vi "SISO-State-Space-Model-01.vi"() -> ()   [LabVIEW 2022 SP3]
uses:
  <vilib>/addons/System Identification/Model Typedefs.llb/si_Bode Magnitude Plot.ctl
  <vilib>/addons/System Identification/Model Typedefs.llb/si_Bode Phase Plot.ctl
  <vilib>/Utility/file.llb/Read Delimited Spreadsheet (DBL).vi
  <vilib>/addons/System Identification/Frequency Domain Estimation.llb/SI Estimate Discrete Transfer Function Model from FRF (SISO Arbitrary).vi
  <vilib>/addons/System Identification/NI_SysID.lvlib
  <vilib>/addons/System Identification/Frequency Domain Estimation.llb/SI Estimate Discrete State-Space Model from FRF (SISO Arbitrary).vi
  <vilib>/Analysis/NI_AALPro.lvlib
  <vilib>/Analysis/6fits.llb/Confidence Interval (Gauss).vi
  <vilib>/Analysis/6fits.llb/Confidence Interval (Power).vi
  <vilib>/Analysis/6fits.llb/Confidence Interval (Log).vi
  <vilib>/Analysis/6fits.llb/Confidence Interval (Exp).vi
  <vilib>/Analysis/6fits.llb/Confidence Interval (Linear).vi
panel:
  out "Bode phase plot":T1
  out "Bode magnitude plot":T2
  in  "freq info":T3={"start frequency"=-1.0, "end frequency"=-1.0, "num of freq bins"=1000, "interval type"=0} {"interval type" items=["logarithmic", "linear"]; "end frequency" format="%.2f"; "start frequency" format="%.2f"}
  in  "orders of transfer function model":cluster{" num order":i32, "den order":i32}={" num order"=1, "den order"=2}
  out "Observed Data and Fitted Curve":cluster{cluster{dbl, "Numeric":dbl}[]}[](graph)
  in  "Data Set":T4(ring)
  in  "Tolerance":dbl=0.0001
  in  "Fitting Method":u16(ring) items=["Least Square", "Least Absolute Residual", "Bisquare"]
  out "Slope Value":dbl format="%#.6g"
  out "Intercept Value":dbl format="%#.6g"
  out "Standard Deviation":dbl
  out "Residue":dbl
  in  "Stop":bool
  in  "Amplitude":string="Amplitude"
  out "Phase Response":cluster{"frequency":dbl[], "amplitude":dbl[]}[](graph)
  out "Magnitude Response":cluster{"frequency":dbl[], "amplitude":dbl[]}[](graph)
  in  "Order":i32=30
  out "Phase":cluster{"Array":dbl[], "Array":dbl[]}(graph) caption="Amplitude [Hz]"
  in  "Skip First N Lines":i32=48
  out "Magnitude":cluster{"Array":dbl[], "Array":dbl[]}(graph) caption="Amplitude [Hz]"
  out "number of rows":i32
  in  "name or relative path":path=path "C:/Users/LAV-UFSC/Documents/LAV - TCC/Dados-Experimentos/25-04/frf_2.txt"
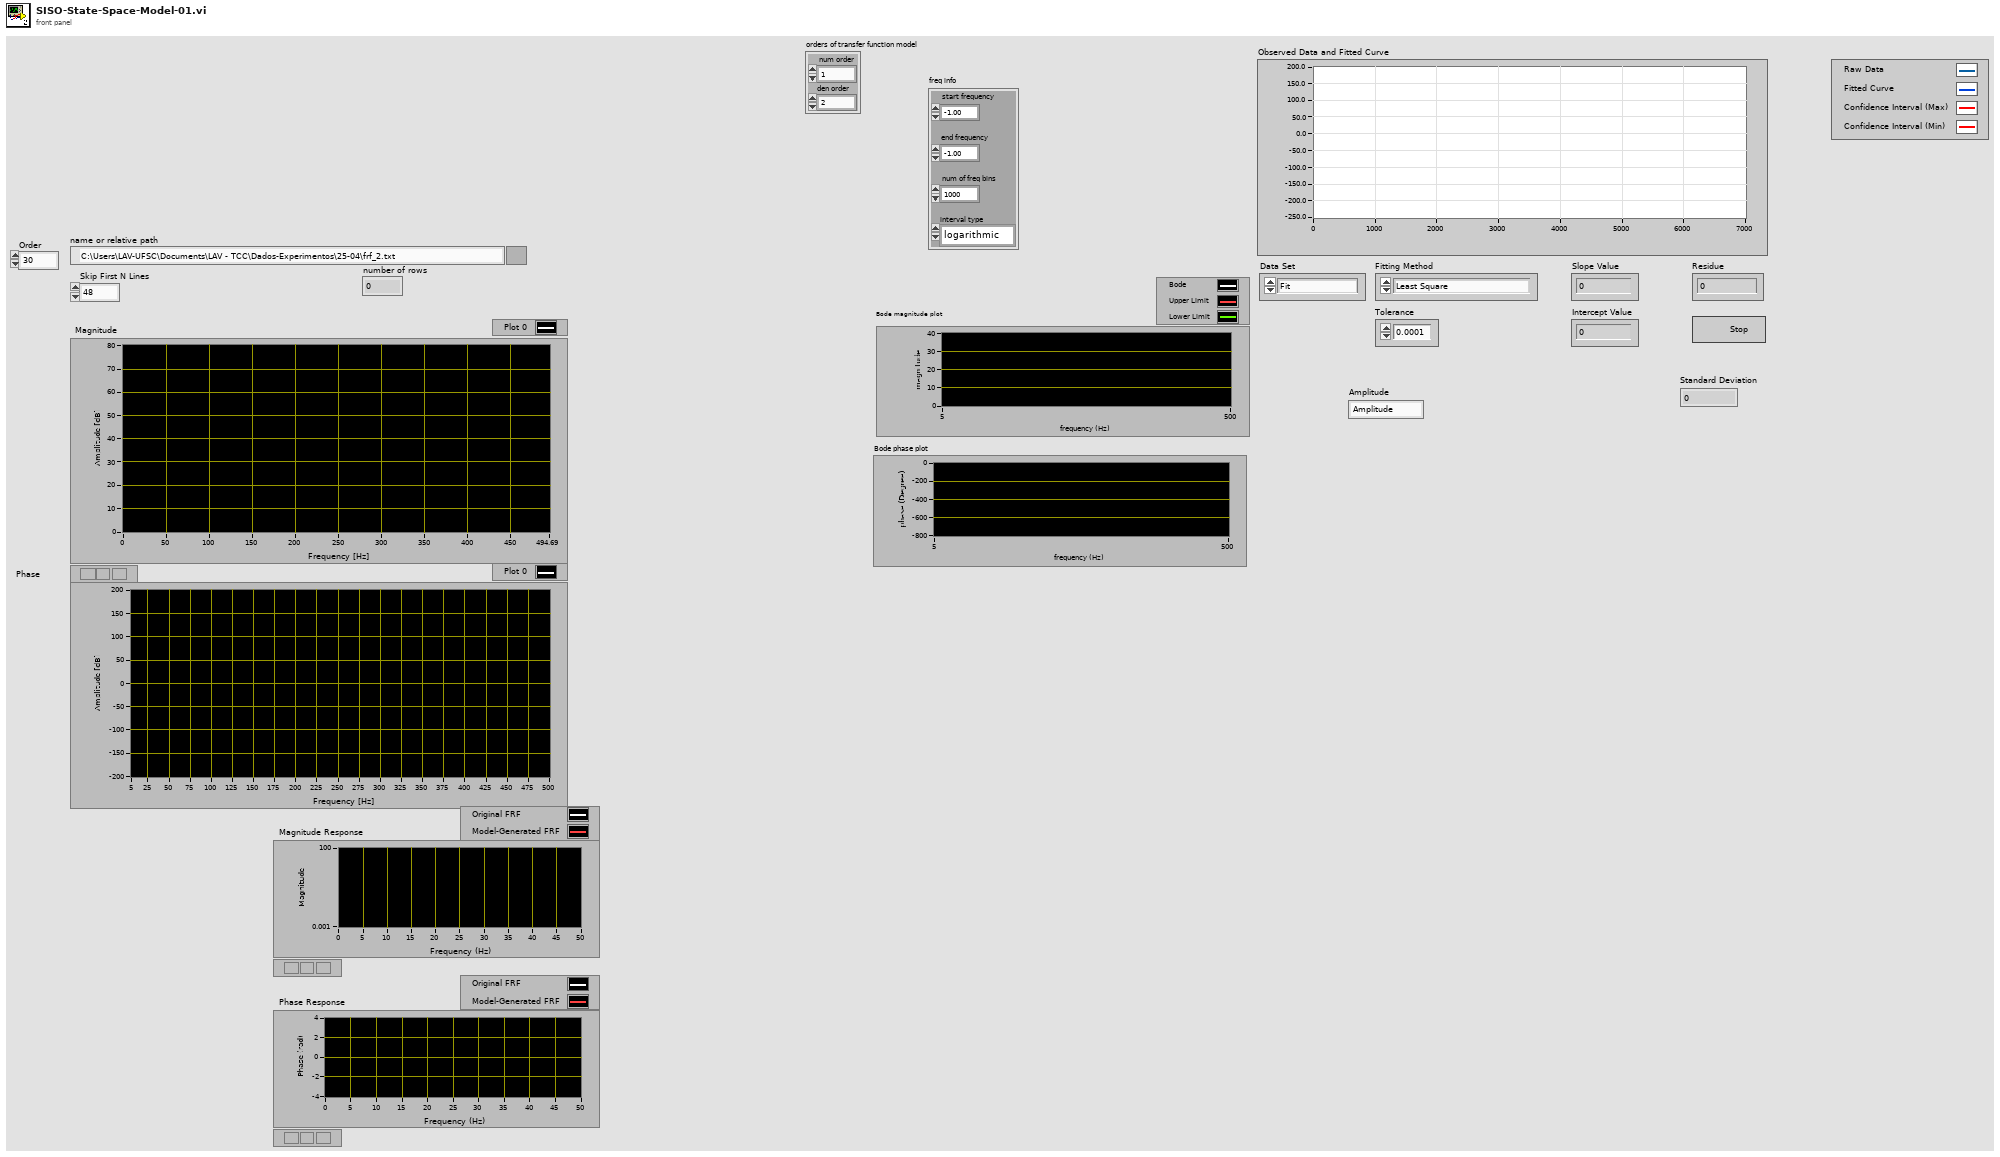
[diagram p1: front panel]
types:
  T1 = typedef "NI_SysID.lvlib/si_Bode Phase Plot.ctl" = cluster{"frequency":dbl[], "amplitude":dbl[]}[]
  T2 = typedef "NI_SysID.lvlib/si_Bode Magnitude Plot.ctl" = cluster{"frequency":dbl[], "amplitude":dbl[]}[]
  T3 = cluster{"start frequency":dbl, "end frequency":dbl, "num of freq bins":i32, "interval type":u16}
  T4 = enum16{"Fit", "Linear", "Exponential", "Power", "Gaussian", "Logarithmic"}
  T5 = typedef "NI_SysID.lvlib/si_generic model.ctl" = cluster{"attributes":cluster{"version":string, "model type":T6, "input names":string[], "output names":string[], "notes":string}, "coefficients":cluster{"A ":dbl[][][], "B":dbl[][][], "F":dbl[][][], "C":dbl[][][], "D":dbl[][][]}, "std deviations":cluster{"A ":dbl[][][], "B":dbl[][][], "F":dbl[][][], "C":dbl[][][], "D":dbl[][][]}, "coefficients covariance":dbl[][][], "noise variance":dbl[][], "fs":dbl, "system info":cluster{"number of inputs":i32, "number of outputs":i32, "A order":i32[][], "B order":i32[][], "F order":i32[][], "C order":i32[][], "D order":i32[][], "Delays":i32[][]}, "kalman gain":dbl[][], "initial state":dbl[], "trans func":cluster{"betas":dbl[], "alphas":dbl[]}[][], "zeros-poles":cluster{"zeros":cdb[], "poles":cdb[], "gain":dbl}[][], "std of trans func":cluster{"betas":dbl[], "alphas":dbl[]}[][], "std of zeros-poles":cluster{"zeros":cdb[], "poles":cdb[], "gain":dbl}[][], "trans func (noise)":cluster{"betas":dbl[], "alphas":dbl[]}[][], "std of trans func (noise)":cluster{"betas":dbl[], "alphas":dbl[]}[][], "zeros-poles (noise)":cluster{"zeros":cdb[], "poles":cdb[], "gain":dbl}[][], "std of zeros-poles (noise)":cluster{"zeros":cdb[], "poles":cdb[], "gain":dbl}[][], "Symbolic State Space Model":cluster{"Symbolic A":string[][], "Symbolic B":string[][], "Symbolic C":string[][], "Symbolic D":string[][], "Symbolic K":string[][], "Symbolic Initial State":string[]}, "delay":dbl[][], "variables":T7, "grey trans func spec":cluster{"orders of TF model":cluster{" num order":i32, "den order":i32}, "# of zeros/poles at origin":cluster{"zeros/poles":u16, "number ":i32}, "delay initial?":bool, "gain initial?":bool}}
  T6 = typedef "NI_SysID.lvlib/SI Model Type.ctl" = u16
  T7 = typedef "NI_SysID.lvlib/si_variables.ctl" = cluster{"name":string, "initial guess":dbl, "upper limit":dbl, "lower limit":dbl, "value":dbl}[]
  T8 = cluster{"frequency":dbl[], "phase (wrapped)":dbl[]}
  T9 = cluster{"frequency":dbl[], "phase (wrapped)":dbl[]}[]
  T10 = cluster{cluster{"Numeric":dbl, "Numeric":dbl}[]}[]
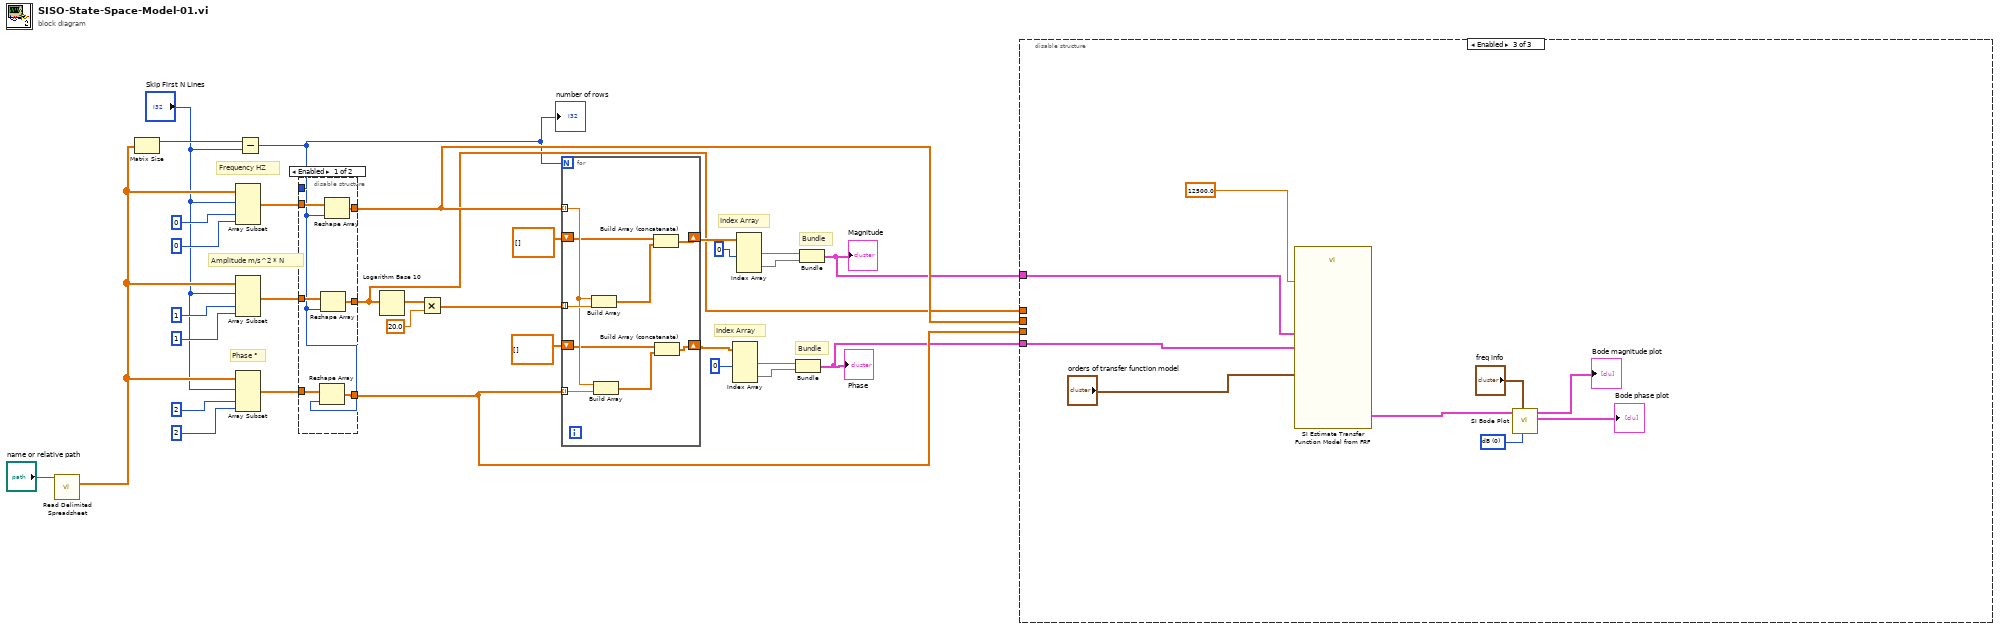
[diagram p0: block diagram]
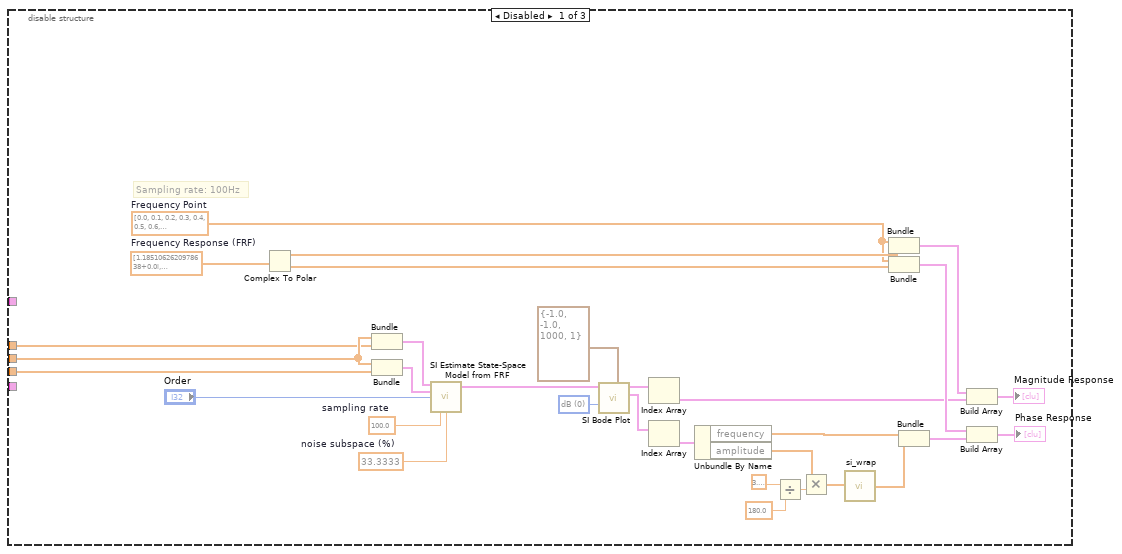
[diagram p2: hidden frame]
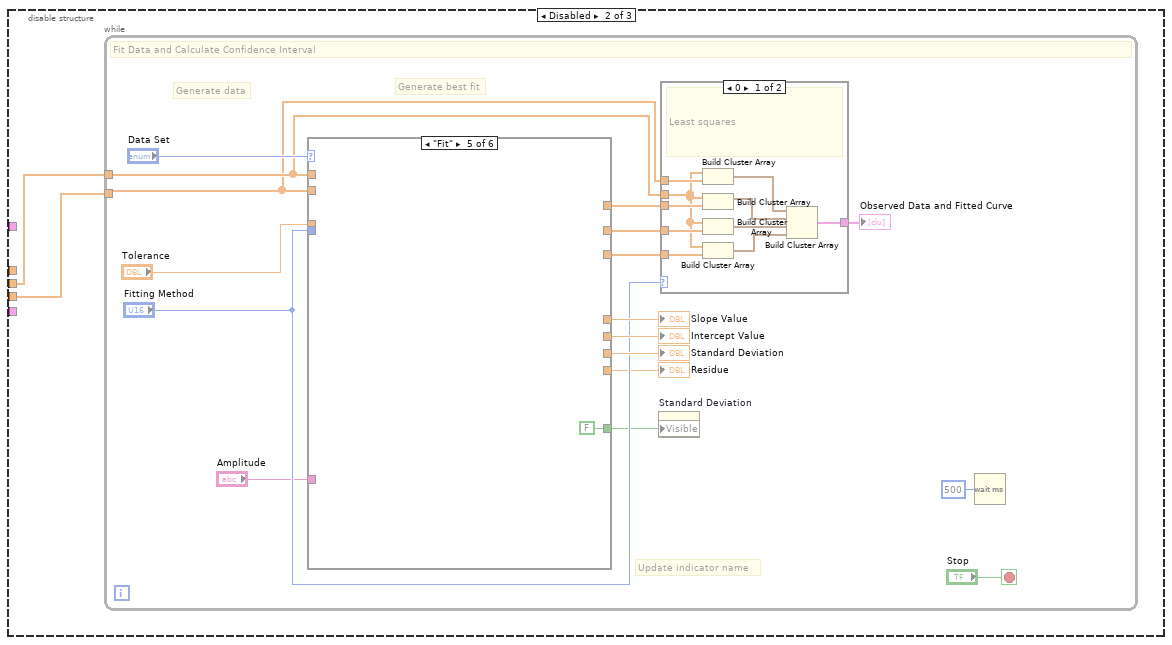
[diagram p3: hidden frame]
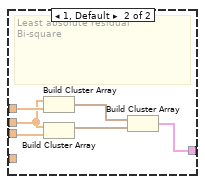
[diagram p4: hidden frame]
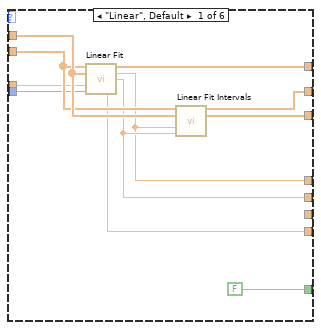
[diagram p5: hidden frame]
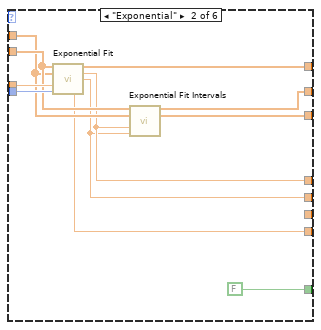
[diagram p6: hidden frame]
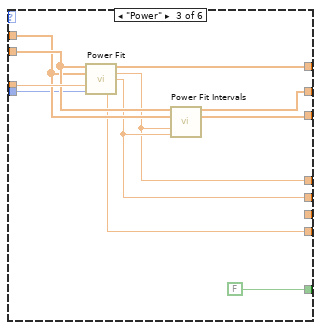
[diagram p7: hidden frame]
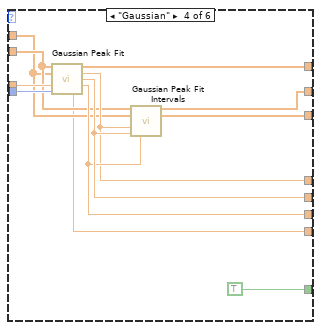
[diagram p8: hidden frame]
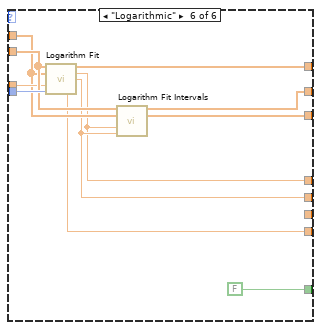
[diagram p9: hidden frame]
diagram:
  # "Index Array"
  # "Bundle"
  # "Index Array"
  # "Bundle"
  # "Phase °"
  # "Amplitude m/s^2 * N"
  # "Frequency HZ"
  n1 = call-poly <vilib>:"Read Delimited Spreadsheet.vi"("file path (dialog if empty)"="name or relative path") -> ("all rows"=w23:dbl[][])  [unwired: 9 in, 5 out]
  n2 = Matrix Size(0:w23) -> (1:w5:i32)  [unwired: 1 out]
  n3 = Array Subset(array=w23, index (row)="Skip First N Lines", index (col)=0 ("column 1"), length (col)=0 ("column N")) -> (w25:dbl[][])  [unwired: 1 in]
  n4 = Array Subset(array=w23, index (row)="Skip First N Lines", index (col)=1 ("column 1"), length (col)=1 ("column N")) -> (w24:dbl[][])  [unwired: 1 in]
  n5 = Array Subset(array=w23, index (row)="Skip First N Lines", index (col)=2 ("column 1"), length (col)=2 ("column N")) -> (w7:dbl[][])  [unwired: 1 in]
  n6 = Subtract(x=w5, y="Skip First N Lines") -> (x-y=w3:i32)
  "number of rows" <- w3
  n7 = disable-structure shown="Enabled" {
    disable-tunnel: w25 -> [w39 w41]
    disable-tunnel: w24 -> [w38 w40]
    disable-tunnel: [w37 w41] -> w9
    disable-tunnel: [w36 w40] -> w8
    disable-tunnel: w3 -> [w34 _]
    disable-tunnel: w7 -> [w35 _]
    disable-tunnel: [w33 _] -> w6
    frame Enabled {
      n8 = Reshape Array(w35, w34) -> (w33:dbl[])
      n9 = Reshape Array(w38, w34) -> (w36:dbl[])
      n10 = Reshape Array(w39, w34) -> (w37:dbl[])
    }
    frame Disabled {
    }
  }
  n11 = Logarithm Base 10(1:w8) -> (0:w16:dbl[])
  n12 = Multiply(x=w16, y=20.0) -> (x*y=w15:dbl[])
  n13 = for {
    N: w3 -> [_]
    tunnel: w9 -> [w48] mode=indexing
    tunnel: w15 -> [w49] mode=indexing
    tunnel: w6 -> [w50] mode=indexing
    shift-right: [w45] -> w18
    shift-left: dbl[][] [] -> [w47]
    shift-right: [w44] -> w10
    shift-left: dbl[][] [] -> [w43]
    n14 = Build Array(w48, w49) -> (w46:dbl[])
    n15 = Build Array(w48, w50) -> (w42:dbl[])
    n16 = Build Array (concatenate)(w47, w46) -> (w45:dbl[][])
    n17 = Build Array (concatenate)(w43, w42) -> (w44:dbl[][])
  }
  n18 = Index Array(array=w10, index (col) #1=0 ("disabled index (col)")) -> (element #1=w11:dbl[], element #2=w12:dbl[])  [unwired: 3 in]
  n19 = Index Array(array=w18, index (col) #1=0 ("disabled index (col)")) -> (element #1=w19:dbl[], element #2=w20:dbl[])  [unwired: 3 in]
  n20 = Bundle(w11, w12) -> (w1:cluster{dbl[], dbl[]})  [unwired: 1 in]
  "Phase" <- w1
  n21 = Bundle(w19, w20) -> (w2:cluster{dbl[], dbl[]})  [unwired: 1 in]
  "Magnitude" <- w2
  n22 = disable-structure shown="Enabled" {
    disable-tunnel: w9 -> [w53 w83 _]
    disable-tunnel: w8 -> [w52 _ _]
    disable-tunnel: w6 -> [w51 w82 _]
    disable-tunnel: w2 -> [_ _ w182]
    disable-tunnel: w1 -> [_ _ w181]
    frame Disabled {
      w56 = dbl[] [0.0, 0.1, 0.2, 0.3, 0.4, 0.5, 0.6, 0.7000000000000001, 0.8, 0.8999999999999999, 1.0, 1.0999999999999999, 1.2, 1.3, 1.4000000000000001, 1.5, 1.6, 1.7000000000000002, 1.7999999999999998, 1.9, 2.0, 2.1, 2.1999999999999997, 2.3, 2.4, 2.5, 2.6, 2.7, 2.8000000000000003, 2.9000000000000004, 3.0, 3.0999999999999996, 3.2, 3.3000000000000003, 3.4000000000000004, 3.5000000000000004, 3.5999999999999996, 3.6999999999999997, 3.8, 3.9, 4.0, 4.1000000000000005, 4.2, 4.3, 4.3999999999999995, 4.5, 4.6, 4.7, 4.8, 4.9, 5.0, 5.1, 5.2, 5.3, 5.4, 5.5, 5.6000000000000005, 5.700000000000001, 5.800000000000001, 5.8999999999999995, 6.0, 6.1, 6.199999999999999, 6.3, 6.4, 6.5, 6.6000000000000005, 6.7, 6.800000000000001, 6.9, 7.000000000000001, 7.1, 7.199999999999999, 7.3, 7.3999999999999995, 7.5, 7.6, 7.7, 7.8, 7.9, 8.0, 8.1, 8.200000000000001, 8.299999999999999, 8.4, 8.500000000000002, 8.6, 8.7, 8.799999999999999, 8.9, 9.0, 9.1, 9.2, 9.3, 9.4, 9.499999999999998, 9.6, 9.700000000000001, 9.8, 9.9, 10.0, 10.100000000000001, 10.2, 10.299999999999999, 10.4, 10.5, 10.6, 10.700000000000001, 10.8, 10.9, 11.0, 11.1, 11.200000000000001, 11.3, 11.400000000000002, 11.5, 11.600000000000001, 11.700000000000001, 11.799999999999999, 11.9, 12.0, 12.1, 12.2, 12.3, 12.399999999999999, 12.5, 12.6, 12.7, 12.8, 12.9, 13.0, 13.100000000000001, 13.200000000000001, 13.3, 13.4, 13.5, 13.600000000000001, 13.700000000000001, 13.8, 13.900000000000002, 14.000000000000002, 14.099999999999998, 14.2, 14.299999999999999, 14.399999999999999, 14.499999999999998, 14.6, 14.7, 14.799999999999999, 14.899999999999999, 15.0, 15.1, 15.2, 15.299999999999999, 15.4, 15.5, 15.6, 15.7, 15.8, 15.9, 16.0, 16.099999999999998, 16.2, 16.3, 16.400000000000002, 16.5, 16.599999999999998, 16.7, 16.8, 16.900000000000002, 17.000000000000004, 17.1, 17.2, 17.299999999999997, 17.4, 17.5, 17.599999999999998, 17.7, 17.8, 17.9, 18.0, 18.099999999999998, 18.2, 18.3, 18.4, 18.500000000000004, 18.6, 18.7, 18.8, 18.9, 18.999999999999996, 19.1, 19.2, 19.3, 19.400000000000002, 19.5, 19.6, 19.7, 19.8, 19.900000000000002, 20.0, 20.1, 20.200000000000003, 20.3, 20.4, 20.499999999999996, 20.599999999999998, 20.7, 20.8, 20.900000000000002, 21.0, 21.099999999999998, 21.2, 21.3, 21.400000000000002, 21.5, 21.6, 21.7, 21.8, 21.9, 22.0, 22.1, 22.2, 22.300000000000004, 22.400000000000002, 22.5, 22.6, 22.7, 22.800000000000004, 22.900000000000002, 23.0, 23.1, 23.200000000000003, 23.299999999999997, 23.400000000000002, 23.5, 23.599999999999998, 23.7, 23.8, 23.9, 24.0, 24.099999999999998, 24.2, 24.3, 24.4, 24.5, 24.6, 24.7, 24.799999999999997, 24.9, 25.0, 25.1, 25.2, 25.3, 25.4, 25.5, 25.6, 25.7, 25.8, 25.900000000000002, 26.0, 26.1, 26.200000000000003, 26.3, 26.400000000000002, 26.5, 26.6, 26.700000000000003, 26.8, 26.900000000000002, 27.0, 27.1, 27.200000000000003, 27.3, 27.400000000000002, 27.500000000000004, 27.6, 27.700000000000003, 27.800000000000004, 27.900000000000002, 28.000000000000004, 28.1, 28.199999999999996, 28.299999999999997, 28.4, 28.499999999999996, 28.599999999999998, 28.7, 28.799999999999997, 28.9, 28.999999999999996, 29.099999999999998, 29.2, 29.299999999999997, 29.4, 29.5, 29.599999999999998, 29.7, 29.799999999999997, 29.9, 30.0, 30.099999999999998, 30.2, 30.3, 30.4, 30.5, 30.599999999999998, 30.7, 30.8, 30.9, 31.0, 31.1, 31.2, 31.3, 31.4, 31.5, 31.6, 31.7, 31.8, 31.900000000000002, 32.0, 32.10000000000001, 32.199999999999996, 32.300000000000004, 32.4, 32.5, 32.6, 32.7, 32.800000000000004, 32.9, 33.0, 33.10000000000001, 33.199999999999996, 33.300000000000004, 33.4, 33.5, 33.6, 33.7, 33.800000000000004, 33.900000000000006, 34.00000000000001, 34.099999999999994, 34.2, 34.300000000000004, 34.4, 34.5, 34.599999999999994, 34.699999999999996, 34.8, 34.9, 35.0, 35.1, 35.199999999999996, 35.3, 35.4, 35.5, 35.6, 35.699999999999996, 35.8, 35.9, 36.0, 36.1, 36.199999999999996, 36.3, 36.4, 36.5, 36.6, 36.7, 36.8, 36.9, 37.00000000000001, 37.099999999999994, 37.2, 37.3, 37.4, 37.5, 37.6, 37.7, 37.8, 37.900000000000006, 37.99999999999999, 38.1, 38.2, 38.3, 38.4, 38.5, 38.6, 38.7, 38.800000000000004, 38.9, 39.0, 39.1, 39.2, 39.300000000000004, 39.4, 39.5, 39.6, 39.7, 39.800000000000004, 39.9, 40.0, 40.1, 40.2, 40.300000000000004, 40.400000000000006, 40.5, 40.6, 40.699999999999996, 40.8, 40.900000000000006, 40.99999999999999, 41.099999999999994, 41.199999999999996, 41.3, 41.4, 41.5, 41.6, 41.699999999999996, 41.800000000000004, 41.89999999999999, 42.0, 42.1, 42.199999999999996, 42.3, 42.4, 42.5, 42.6, 42.699999999999996, 42.800000000000004, 42.89999999999999, 43.0, 43.1, 43.2, 43.3, 43.4, 43.5, 43.6, 43.7, 43.8, 43.9, 44.0, 44.1, 44.2, 44.3, 44.4, 44.5, 44.60000000000001, 44.699999999999996, 44.800000000000004, 44.9, 45.0, 45.1, 45.2, 45.300000000000004, 45.4, 45.5, 45.60000000000001, 45.699999999999996, 45.800000000000004, 45.9, 46.0, 46.1, 46.2, 46.300000000000004, 46.400000000000006, 46.50000000000001, 46.599999999999994, 46.7, 46.800000000000004, 46.9, 47.0, 47.099999999999994, 47.199999999999996, 47.3, 47.4, 47.5, 47.6, 47.699999999999996, 47.8, 47.9, 48.0, 48.1, 48.199999999999996, 48.3, 48.4, 48.5, 48.6, 48.699999999999996, 48.8, 48.9, 49.0, 49.1, 49.2, 49.3, 49.4, 49.50000000000001, 49.599999999999994, 49.7, 49.8, 49.9]  # Frequency Point
      w59 = 100.0  # sampling rate
      w75 = u16 0 items=["dB", "linear"] ("magnitude unit")
      w78 = 33.3333  # noise subspace (%)
      w63 = cdb[] [1.1851062620978638+0.0i, -0.0064518026653783+0.0025726850415727916i, -0.012607604818783473+0.003207018853718229i, -0.009618842696386493+0.012651488302640181i, 0.01036812842121885+0.01576750539476137i, -0.006701196352090295+0.023078030896190944i, 0.0031494580732113757+0.011917589751699825i, 0.02131555234082974+0.02449029613261991i, 0.023587501187049657+0.006149022530173854i, 0.01978378018943642+0.002234698050171249i, 0.01717628850778748+0.0002602315772577525i, 0.015384045067266153-0.00039294302226473144i, 0.014822378453775938-0.00012537748100161078i, 0.015180637747176285-0.0007378646396296322i, 0.015067354568189525-0.001379781819394797i, 0.015181419189380665-0.001755285678617077i, 0.01550838054649081-0.0020975756927374203i, 0.01600105325390315-0.002373721749134176i, 0.016824548679866193-0.0027711005869251923i, 0.018000843454816815-0.0031817936414539213i, 0.019730440657361212-0.0037278521294683655i, 0.02240944103313504-0.004310692925640184i, 0.02746010002228881-0.005346725427408711i, 0.03920524718129086-0.008303880279410859i, 0.09157465910161641-0.034762590833219434i, -0.06958205145098131-0.017320782246361965i, -0.018151319127681306-0.004559243237991757i, -0.006926581493980713-0.003970897442287139i, -0.0018531407117842623-0.004100879044493743i, 0.0010553897015824767-0.004306730133319881i, 0.0030441040480015885-0.004599613515188549i, 0.004507584124527005-0.004920197389460303i, 0.005634238355491219-0.0052644926869226056i, 0.0065335906424258735-0.0055664443920206905i, 0.007382608970996207-0.005871236573027153i, 0.008162846875869656-0.006197197568251888i, 0.008900544323409986-0.006572286038752292i, 0.009586725393629161-0.006924474855990149i, 0.01029706022041439-0.007352882656280581i, 0.010912132519657938-0.0077407181195691815i, 0.01164760540663557-0.008175459109898043i, 0.012378193669938477-0.008645468807936499i, 0.013204523735403864-0.009244299222905133i, 0.01392005532854377-0.009733217946323008i, 0.014743325651913552-0.010299683559216413i, 0.015673402559531483-0.010918390158245816i, 0.016629357381695766-0.01162240461332872i, 0.01770014159242484-0.012353733623156738i, 0.018889522873172353-0.013160139743079675i, 0.020193013205897944-0.014097171537701491i, 0.02167466057377768-0.015135347539476169i, 0.023285735832060502-0.0163323450064265i, 0.024966347214093465-0.017690112154298377i, 0.027117811934750508-0.01896025090143955i, 0.029577122829468686-0.02061879525817235i, 0.032506903464983736-0.022726773799331294i, 0.035639413572987076-0.025165307477286774i, 0.03843789620362705-0.027466276954241257i, 0.04734237715269786-0.03188988299374438i, 0.05270294065637172-0.03651717591340596i, 0.061158305339231424-0.042114180550888995i, 0.07345709787423968-0.050308381411654855i, 0.09117057953286974-0.06259491768084782i, 0.11917282869427182-0.08252093732675894i, 0.17333368770506513-0.12091501033347161i, 0.3047661910228993-0.21831879418734923i, 1.2394474198755623-1.0968606175963285i, -0.5865484070751298+0.35583474020463246i, -0.24038723384237748+0.15423284588706898i, -0.15204328331809236+0.09830654311233951i, -0.11161145970602362+0.07252157835471236i, -0.08802455635727474+0.05736143449636372i, -0.07280418072887075+0.04723738623076344i, -0.06225591953355748+0.04021220489948363i, -0.054438386346396125+0.03492381178789762i, -0.048331996342868104+0.030906552043696838i, -0.04359533762072471+0.027698875323963732i, -0.039543034189082046+0.025067544235121687i, -0.03623839725113517+0.02277579705128849i, -0.03352897312192441+0.02082091274597516i, -0.031171987929296877+0.01919122506168922i, -0.029111692084308315+0.01775462759345584i, -0.027359238356856917+0.016536691962917585i, -0.02571303870219197+0.015379498397177931i, -0.024278231177018363+0.01437521593278256i, -0.02292607808601912+0.013386000810043017i, -0.02184298285375185+0.012564730887562953i, -0.020745621870632846+0.011776029776881745i, -0.01977842160143003+0.011017397504090339i, -0.018866859694951547+0.010313297815371898i, -0.018036195541260985+0.00963679550960992i, -0.017348553926634234+0.00926826296043663i, -0.016507761808191378+0.008575149293524322i, -0.015805667721324048+0.007988731579220443i, -0.01513069714413463+0.007437750583756714i, -0.014473208817906293+0.006934578303479637i, -0.013885122177934162+0.006419329201559824i, -0.013288024532429088+0.005892506425437705i, -0.01269052331332068+0.005398821944319895i, -0.012131775871433992+0.0049096038828279585i, -0.011555745063734545+0.004414593737158132i, -0.01100526564571187+0.00391733471405611i, -0.010478465655873207+0.003437106242788574i, -0.009922080860405722+0.0029165232594384597i, -0.009341743109223817+0.002398263174020962i, -0.008779429645472977+0.0019116883740585742i, -0.008100124976172018+0.001143242662760016i, -0.007559780672320459+0.0006051924504366104i, -0.006979544157546345-4.632309100622806e-05i, -0.0063225563431855885-0.0006777586711666256i, -0.0056217518608119126-0.0014119358451113962i, -0.004859677260638813-0.0022053724493177763i, -0.004117410616594437-0.002968491887805332i, -0.0032050356007870856-0.00390622960733713i, -0.002245551837881647-0.004993876404198736i, -0.0011769500872260323-0.006222632156630903i, 0.00013913299396588172-0.007540905588148345i, 0.001729523446570073-0.009233708902186805i, 0.0038127829113796664-0.011588063438628025i, 0.007065761619635297-0.015412534657897981i, 0.02309946711308761-0.0422580109848221i, 0.0006360076936776966-0.009732543555401263i, 0.006925879005686296-0.016080537335524087i, 0.011455724989926218-0.020965201932091393i, 0.01673943125961907-0.02689261243352685i, 0.02322020815644174-0.03464326710944107i, 0.03237615501767741-0.045815230565381i, 0.047754428322406714-0.06377671319824867i, 0.07723109546651528-0.09970099042363575i, 0.15602839919262262-0.20460347563411216i, 0.702025222213564-2.5806510916803522i, -0.24286515087690305+0.24666920608302914i, -0.11990796183857494+0.123728409963007i, -0.08266868294935444+0.0867714989105894i, -0.0644639527313388+0.06642445159367304i, -0.05385640230628613+0.054708910705290305i, -0.04684286838309362+0.04676964523960857i, -0.041744126661271835+0.04118252809014438i, -0.03808839487778581+0.0370317514452557i, -0.035109802353784164+0.03379976853899189i, -0.03274377584261456+0.031111804336391744i, -0.030875737220831524+0.02894845386575411i, -0.029336209755429127+0.027149404580302603i, -0.028012999514629922+0.025633996374394622i, -0.026852599668989768+0.024337188459138275i, -0.025875583918032876+0.023213623118691223i, -0.02494761237756119+0.022229782857838096i, -0.024192352741507113+0.021369155703879362i, -0.023465218431077937+0.020618427954712908i, -0.02277947057437749+0.019779179587343584i, -0.022297611471445183+0.019155619538662513i, -0.021765369041863446+0.018596554709697677i, -0.021316102463962143+0.018061854602161413i, -0.020876011042291948+0.01758258173627944i, -0.02052326090267134+0.017032726267984556i, -0.0201675683848129+0.017040774723682844i, -0.019774992633079396+0.016545813153028062i, -0.01941458931541117+0.01612119543167552i, -0.019163511387085427+0.015786300345727117i, -0.018902418578943425+0.015483166585782871i, -0.01861482157508898+0.015254029049032346i, -0.018360379150823336+0.014980890139128407i, -0.018116460912850164+0.014734244272274556i, -0.01789029524575753+0.01447168658169178i, -0.017725736953084978+0.014239345916774261i, -0.017497676010540524+0.014087972415218373i, -0.01725844880177687+0.013901022110524413i, -0.017076182672314064+0.013727079313619966i, -0.016896796687089162+0.013528555272605242i, -0.016748992679583605+0.013456138987413283i, -0.016578483253933813+0.013293284062702321i, -0.016376372987491256+0.013147638249212114i, -0.01614264925284271+0.013024998927372456i, -0.01600568166688934+0.012901838094904566i, -0.015807624831206256+0.012824352838935175i, -0.015639075493606807+0.012660101901782739i, -0.015465709377444962+0.012590201131378898i, -0.015227625490309295+0.012582152337288722i, -0.015254471157434703+0.012176641498269214i, -0.01493234852792234+0.0122212118525919i, -0.014709072767747694+0.012208083000746486i, -0.014578525499969743+0.012186270910164367i, -0.01434227442859985+0.01204968869492709i, -0.014081190559571789+0.012060307227401864i, -0.013787346518497579+0.012147133944982267i, -0.013285184945553613+0.012113855451467936i, -0.012624934149701313+0.012170357198379174i, -0.011723735438208892+0.012316028693806713i, -0.00893356538945381+0.013027065417604318i, -0.02663109782192257-0.047170954269533404i, -0.01810832509617651+0.008954547004716462i, -0.01579639562597485+0.010137072510982769i, -0.014795271797106633+0.01027712371527519i, -0.014400474752718153+0.010212712627301635i, -0.013932949571262324+0.01010320534450086i, -0.014132634314570899+0.009581541373580159i, -0.017536762016596708+0.0069543483467837i, -0.009736206179732155+0.014645172069526504i, -0.010505908314798508+0.012299322090492035i, -0.010341312842947445+0.011753609898786706i, -0.00988598466589429+0.01157770810572586i, -0.009411696121926705+0.011359726989302892i, -0.00875532249967349+0.011324051942312065i, -0.007936425435768743+0.011202034836974076i, -0.007050451097696457+0.011223311722893743i, -0.005863652357367224+0.011139634673309503i, -0.00449848809790352+0.0110884934570911i, -0.0028158172073191293+0.011006833759364535i, -0.0005226052513086101+0.011202469182794956i, 0.002782267921458836+0.011159163675249738i, 0.0072614450592533575+0.010927388728578727i, 0.013982572428838023+0.010377555910718386i, 0.025476778940428834+0.00893070943559345i, 0.0483285285259233+0.004253051083257392i, 0.1168980226604867-0.02658085958106237i, -0.16425773658232637-0.3575435229200716i, -0.12300407015334336-0.02200378107738455i, -0.0772262751448223-0.0007334751973584854i, -0.05922054701969503+0.004681163686272562i, -0.049727181823364816+0.00672672643501677i, -0.043968813001020686+0.007866871416455975i, -0.0401940256987709+0.008452966111921895i, -0.03721251849240739+0.008912710487055275i, -0.03526271160047395+0.009241766395073885i, -0.03362503438573791+0.00959378995604317i, -0.03227116417541715+0.009719066813376366i, -0.03114981232875083+0.009832523356182307i, -0.030342563823068734+0.00999871505369641i, -0.029607260370542246+0.010118105941478358i, -0.02894011174358598+0.010220500516714134i, -0.02836905479042695+0.010230166116009107i, -0.028111259764222397+0.010521484205230995i, -0.027616997072147494+0.010592390688970882i, -0.027306120037966883+0.010451115735020817i, -0.02700797458497407+0.010778389959989636i, -0.02683636161001159+0.010875872706183088i, -0.026591555375079436+0.010962540753025796i, -0.026271460142623854+0.010955866409394402i, -0.02606254429242126+0.011081794022067019i, -0.025997115825946878+0.01141588697895282i, -0.025479671748506516+0.01123888276113661i, -0.026096596658740805+0.011424696612699705i, -0.02567172960031331+0.011531086420113513i, -0.025663832960096895+0.011630616719125493i, -0.025591306824424297+0.011414900129862276i, -0.025446639165630145+0.01157422770690568i, -0.025477135936805517+0.011658433257775904i, -0.02516842244143213+0.012263716625637643i, -0.025272216333820548+0.012025840919992443i, -0.025196482561465193+0.012033825207672023i, -0.02519364940774847+0.012170105276165617i, -0.024797459711286465+0.012155780138595789i, -0.02481140006036918+0.012021290651168942i, -0.025207053878347326+0.01229534716951i, -0.02514235504086008+0.01237683063238723i, -0.025379849960426533+0.012283049031112353i, -0.026091499909544333+0.012353045392986295i, -0.025455292225407707+0.013349964593983145i, -0.025401920713673597+0.013122121177643534i, -0.02633582279225662+0.013800359063361542i, -0.03224104221597815+0.021221595235261598i, -0.02099454334504905+0.011940612743804533i, -0.02238641015391949+0.012394651773803845i, -0.02288452239508068+0.012802284625749456i, -0.022422001380860906+0.012777075614793064i, -0.021604776357190356+0.012138346914786826i, -0.01995546960998687+0.011656573814374654i, -0.015717545487735664+0.009317096441930668i, -0.0106655635241003-0.07049745737526486i, -0.038853204960803585+0.014845351084125515i, -0.03306680412717024+0.01673061080756434i, -0.029838603100755312+0.015790660648230145i, -0.029088931793771883+0.015165020666047179i, -0.028391228679324632+0.015113079677349274i, -0.028455898830227283+0.015237730631685462i, -0.028520622448425056+0.015363807093416787i, -0.028212009863055176+0.015268739262564671i, -0.028334944807018033+0.015028652184856587i, -0.028410538148829455+0.014590662195885368i, -0.029362611136030697+0.014429578259018298i, -0.030438669003709732+0.0180238234136009i, -0.029281982197537137+0.0175969232208617i, -0.028244373323260692+0.016036142701148195i, -0.028566807532370904+0.01579429999967927i, -0.028660542407730746+0.015367899964962479i, -0.029489024182213743+0.015644280342436936i, -0.029360792301555094+0.01574049375361208i, -0.02947807852388983+0.016040864633802596i, -0.030083286036347665+0.01574088508975384i, -0.030321550381243793+0.015691244561971813i, -0.03099114170709679+0.015725594820101444i, -0.031152921321029356+0.01556472750276732i, -0.03164684358843067+0.015563698918118813i, -0.03232007242983021+0.015365984127137088i, -0.033823427369610914+0.015338706145773274i, -0.03335624495271358+0.015440942450366537i, -0.03461926419073457+0.015223869849052798i, -0.03587964691312888+0.015481010778508036i, -0.03598744078663133+0.014812216898102469i, -0.03745119804944053+0.014737856207764308i, -0.03862002829193308+0.014472392038582646i, -0.04004075162752458+0.014614733107109187i, -0.04095768491211258+0.014502720626531438i, -0.042819893290034564+0.013855338247515572i, -0.044316284254509+0.013415841065300013i, -0.046921878539912594+0.012406805150144369i, -0.05001673808196269+0.01215944146221149i, -0.05265532063132224+0.011202001119961775i, -0.05613628573733946+0.010987872519108087i, -0.06064959824922869+0.008736653287743909i, -0.06652836238231719+0.007696096549202205i, -0.07463889329299998+0.005476773612202289i, -0.08462869699657131+0.0032725461853484543i, -0.09687479547967155-0.0001744170355132446i, -0.11664084614693647-0.0031114857672218457i, -0.14751264852355667-0.011421090643618981i, -0.205982046047984-0.02133118351564309i, -0.33795025573352677-0.03358963338617035i, -0.9063287492533795+0.14606115311331327i, 0.6279191565490204+0.7030716779036652i, 0.2813716439495064+0.19839094666679222i, 0.17626977452958453+0.12066155568974275i, 0.13049000230365024+0.09408940070650465i, 0.10167146188348379+0.08120391742002485i, 0.08190244063787726+0.06857758921153616i, 0.0697936442240128+0.06459378800221868i, 0.06364506147239479+0.060961900491569236i, 0.05611668335318596+0.059338833245702785i, 0.05277820059468819+0.0571082749246886i, 0.04848191905569953+0.0545283839635904i, 0.04683615410387925+0.053200995929388796i, 0.044436835571359766+0.05101227329160627i, 0.038889875766875616+0.04954747113978973i, 0.037997206537458576+0.05196753551116505i, 0.04408855457397984+0.05054422497274221i, 0.040201362478509556+0.04916957496484516i, 0.04094306380497747+0.04637493746517539i, 0.03812699969576464+0.04842102534235498i, 0.03809903374632165+0.04595013798455146i, 0.037515079345265+0.04794290789212221i, 0.037427023307488774+0.047909327001104535i, 0.03877259309665187+0.04701969868819734i, 0.04134855504502366+0.048183573192709835i, 0.04104287330975697+0.04701242446708746i, 0.041122630052246346+0.04469247716187142i, 0.04422060573168718+0.04759837856393825i, 0.04471687510187678+0.04537061025653618i, 0.045775187128991264+0.047617736640706i, 0.045215361615891014+0.046176377831687605i, 0.0478008761390823+0.0457340967581396i, 0.05031360079171147+0.045173776631442786i, 0.04965296996292676+0.04496288387303094i, 0.05477466289014371+0.04500414304551632i, 0.05809053332189797+0.04589892668777576i, 0.06071249828138983+0.04359088533380899i, 0.05999224409389354+0.04637339488820667i, 0.0666926341357703+0.04697748344950991i, 0.07020923578322584+0.04274743551006358i, 0.07683686670885338+0.04460141386690349i, 0.0838196236745648+0.04385822397738498i, 0.10213268952949699+0.03908539945362726i, 0.07110021300498014-0.06879235131832516i, 0.04883133797232632+0.029886719082286847i, 0.0654373091428696+0.03838775176484284i, 0.0739012188353821+0.03938453227603243i, 0.07969305717487117+0.040142063127621905i, 0.08738012666280744+0.04157516456047993i, 0.09255004622375866+0.041252425790066376i, 0.10137485126497288+0.039845987452256384i, 0.10621136061992248+0.038353824643161255i, 0.11536506181674826+0.0383923090023813i, 0.12266364967375154+0.03959128877914002i, 0.13102372037491938+0.034590942949834134i, 0.14051918266422542+0.0352934985189588i, 0.1546188856500707+0.035252135737300606i, 0.16565903651793307+0.03207263562436886i, 0.18159920879597247+0.029969483942602577i, 0.19766332330696837+0.02642895210384132i, 0.21667631274195898+0.022712551279680967i, 0.24301823639088047+0.014515525051070717i, 0.2760465773709473+0.010993623216016145i, 0.3175332849717554+0.009767742299805272i, 0.38034847148433826-0.00703875284133228i, 0.4649181872120056-0.030888653867075518i, 0.6290846495221555-0.07846955783133053i, 0.9665316380107727-0.24545725583552364i, 2.1611003382163583-1.9726244241471225i, -1.5096492732919826-0.30793490934620693i, -0.534078548185434+0.05397647286606849i, -0.239987988259347+0.0781868296647591i, -0.09035833457501032+0.08650029326051373i, 0.016087000582333092+0.08669826197485196i, 0.1078814139496873+0.0838546466723474i, 0.20192634821835886+0.07988152471895156i, 0.30017559926334414+0.07394750972555426i, 0.43018834733902483+0.06585293583946461i, 0.6224179501065513+0.04183550756991821i, 0.9287523376273658-0.0032381268857119417i, 1.550276252545853-0.17555843223654052i, 3.3357498819240496-1.4688385369234915i, -3.514858817326108-5.230506262069414i, -2.2612494762379893-0.7710896596912319i, -1.4432048800801238-0.2807144107919505i, -1.060703773510725-0.1322984636322939i, -0.8405124651708406-0.06008343985908217i, -0.7100567277042613-0.04338797944753257i, -0.6204155295804015-0.02378442925892118i, -0.5602434761393283-0.006464400630936139i, -0.5077068799194835+0.004081981051056797i, -0.4694322239166599+0.012878062067518962i, -0.43431219630846934+0.011003582747388248i, -0.4035031616351226+0.010531470590714215i, -0.3835955589193439+0.012772660232411298i, -0.3690180377153583+0.02523070229896018i, -0.34716875488403764+0.021114312980615953i, -0.3390401524368996+0.021198703649610153i, -0.32585654894124894+0.022918268425278453i, -0.31494123402427526+0.02647048234886394i, -0.3076877231655502+0.02305441770204591i, -0.29952645847590786+0.025145541236613556i, -0.2933303589808096+0.028144859189222386i, -0.2819304941015544+0.027291657422122532i, -0.28311974343598595+0.029477112759538966i, -0.279328602685487+0.03225233850984356i, -0.26915290207883863+0.03072965177560076i, -0.26788763100616414+0.034362341165364414i, -0.2628105320342859+0.030802626927533022i, -0.26046950569343286+0.02855830195843339i, -0.25891487872812713+0.03234411986000692i, -0.2566389689050609+0.029571294812737056i, -0.25793724434177034+0.029532202908129346i, -0.25233336129532496+0.03151343361562819i, -0.2539698529846198+0.027703151674247164i, -0.2575505595902652+0.029549034044811868i, -0.25552450805441995+0.027190711032612936i, -0.25842243333824505+0.027440808958733708i, -0.2593271371964942+0.028038101516070585i, -0.26341959708267865+0.03195963756296694i, -0.2664251892259522+0.030535239480726274i, -0.2742395747148752+0.031006224359935608i, -0.27397114683153284+0.024455840383848973i, -0.28297503604123425+0.023104602510310743i, -0.29138274892703264+0.016792109006281534i, -0.3060197225780449+0.019128521951306016i, -0.31938733588989393+0.01955571264718271i, -0.34183230469585385+0.028147793978529907i, -0.3635741846694713+0.005487272876002642i, -0.33166039049809287-0.04516198465484001i, -1.1294291146813118-0.2703225792553899i, -1.678640584001047+0.34386543594083574i, 0.9771010634716537+1.3438948008338811i, 0.3353968581274427+0.2939650054726795i, 0.12918009008942002+0.16138859257975022i, 0.03257090949908212+0.11805058309002084i, -0.01463329919279009+0.10009359510035669i, -0.046584400541191506+0.07829583422017537i, -0.06855654284197191+0.06875776275795321i, -0.08641823798872347+0.05515424819435116i, -0.10222938391946511+0.058803809816727996i, -0.10801633342330681+0.06040447306326302i, -0.1213106201585682+0.05362786204858745i, -0.13115797642156082+0.05052992659088881i, -0.13181032685407224+0.046558271465801895i, -0.13691228132064545+0.04388875299707787i, -0.14196820276718236+0.04311161753616811i, -0.15121449848519986+0.038823787236868135i, -0.15812472398843985+0.045266963987527935i, -0.1547807552592045+0.0367906185562901i, -0.16471646962353623+0.03441320521322836i, -0.1981230356594557+0.026299317691644553i, -0.11459749365225567+0.06541678012659984i, -0.14022220239892202+0.039870706099843736i, -0.14894096445448632+0.02952489005825645i, -0.1556339973147702+0.02342466238147137i, -0.15600519530376264+0.020527850487743325i, -0.15274800496880955+0.006013012916675594i, -0.15625455657261086-0.0334360428554825i, -0.27793864051545514+0.07234485910165248i, -0.19307261404837708+0.06217077469160718i, -0.1868690300778103+0.04211149656741515i, -0.18139966914379224+0.04159171270142144i, -0.17940255606221503+0.034816848574879294i, -0.18080372813277776+0.031203638990863494i, -0.18026254800181146+0.026224203637698885i, -0.18207381814381227+0.02850587224147602i, -0.1835608536038278+0.021538164452991313i, -0.18296545891705254+0.02082116974648798i, -0.18496213948640533+0.01993198105947581i, -0.18484895613974192+0.01793517206815012i, -0.18557991322944248+0.017458854798411277i, -0.1892888955910731+0.01366497136822988i, -0.18889188900318704+0.012444178382536336i, -0.18660275746973376+0.00954130949741811i, -0.19226275347272376+0.009897399047977545i, -0.1926173462238859+0.009500994900371566i, -0.19167616727310516+0.00592668625480675i, -0.18959681834618905+0.004406929511508019i, -0.19100113172571379+0.005261862268595865i, -0.1905007762094034+0.0024417640617471854i, -0.193083783715602-0.0010004800850007846i]  # Frequency Response (FRF)
      # "Sampling rate: 100Hz"
      n23 = Complex To Polar(r * e^(i*theta)=w63) -> (r=w61:dbl[], theta=w60:dbl[])
      n24 = Bundle("all rows"=w53, "all rows"=w52) -> (w81:cluster{"all rows":dbl[], "all rows":dbl[]})  [unwired: 1 out]
      n25 = Bundle("all rows"=w53, "all rows"=w51) -> (w80:cluster{"all rows":dbl[], "all rows":dbl[]})  [unwired: 1 out]
      n26 = call-poly <vilib>:"SI Estimate State-Space Model from FRF.vi"("FRF magnitude"=w81, "FRF phase"=w80, "number of states"="Order", "sampling rate (Hz)"=w59, "noise subspace (%)"=w78) -> ("system model out"=w77:T5)  [unwired: 3 in, 7 out]
      n27 = call <vilib>:"SI Bode Plot.vi"("magnitude unit"=w75, "freq info"=T3 {"start frequency"=-1.0, "end frequency"=-1.0, "num of freq bins"=1000, "interval type"=1}, "system model"=w77) -> ("Bode phase plot"=w67:T1, "Bode magnitude plot"=w64:T2)  [unwired: 4 in, 3 out]
      n28 = Index Array(array=w64) -> (element=w57:cluster{"frequency":dbl[], "amplitude":dbl[]})  [unwired: 1 in]
      n29 = Index Array(array=w67) -> (element=w69:cluster{"frequency":dbl[], "amplitude":dbl[]})  [unwired: 1 in]
      n30 = Unbundle By Name(w69) -> ("frequency"=w58:dbl[], "amplitude"=w68:dbl[])
      n31 = Divide(x=3.141592653589793, y=180.0 ("x")) -> (x/y=w70:dbl)
      n32 = Multiply(x=w68, y=w70) -> (x*y=w72:dbl[])
      n33 = call <vilib>:"si_wrap.vi"("phase (upwrapped)"=w72) -> ("phase (wrapped)"=w66:dbl[])
      n34 = Bundle("Frequency Point"=w56, w61) -> (w74:cluster{"Frequency Point":dbl[], dbl[]})  [unwired: 1 out]
      n35 = Bundle("Frequency Point"=w56, w60) -> (w73:cluster{"Frequency Point":dbl[], dbl[]})  [unwired: 1 out]
      n36 = Bundle("frequency"=w58, "phase (wrapped)"=w66) -> (w65:T8)  [unwired: 1 out]
      n37 = Build Array(w74, w57) -> (→"Magnitude Response":cluster{"frequency":dbl[], "amplitude":dbl[]}[])
      n38 = Build Array(w73, w65) -> (→"Phase Response":T9)
    }
    frame Disabled {
      n39 = while {
        tunnel: w83 -> [w85]
        tunnel: w82 -> [w84]
        stop <- "Stop" stop-if-true
        # "Update indicator name"
        # "Generate best fit"
        # "Generate data"
        # "Fit Data and Calculate Confidence Interval"
        n40 = case shown="\"Fit\"" "Data Set" {
          tunnel: [w127 w132 w146 w158 _ w171] -> w97
          tunnel: [w126 w133 w144 w159 _ w173] -> w99
          tunnel: [w125 w134 w145 w160 _ w172] -> w98
          tunnel: w85 -> [w124 w135 w147 w152 _ w167]
          tunnel: w84 -> [w123 w136 w148 w153 _ w169]
          tunnel: "Tolerance" -> [w122 w138 w149 w161 _ w168]
          tunnel: "Fitting Method" -> [w121 w137 w143 w157 _ w170]
          tunnel: [w120 w130 w142 w156 _ w166] -> w95
          tunnel: [w118 w131 w141 w154 _ w165] -> w96
          tunnel: [_ _ _ w155 _ _] -> w94
          tunnel: [w119 w129 w140 w151 _ w164] -> w90
          tunnel: [FALSE ("Visible") FALSE ("Visible") FALSE ("Visible") TRUE ("Visible") FALSE ("Visible") FALSE ("Visible")] -> w87
          tunnel: "Amplitude" -> [_ _ _ _ _ _]
          frame "Linear", Default {
            n41 = call <vilib>:"Linear Fit.vi"("Y"=w123, "X"=w124, "tolerance"=w122, "method"=w121) -> ("Best Linear Fit"=w127:dbl[], "slope"=w118:dbl, "intercept"=w120:dbl, "residue"=w119:dbl)  [unwired: 7 in, 1 out]
            n42 = call-poly <vilib>:"Linear Fit Intervals.vi"("Y"=w123, "X"=w124, "slope"=w118, "intercept"=w120) -> ("Upper Bound"=w125:dbl[], "Lower Bound"=w126:dbl[])  [unwired: 7 in, 3 out]
          }
          frame "Exponential" {
            n43 = call <vilib>:"Exponential Fit.vi"("Y"=w136, "X"=w135, "tolerance"=w138, "method"=w137) -> ("Best Exponential Fit"=w132:dbl[], "amplitude"=w131:dbl, "damping"=w130:dbl, "residue"=w129:dbl)  [unwired: 6 in, 2 out]
            n44 = call-poly <vilib>:"Exponential Fit Intervals.vi"("Y"=w136, "X"=w135, "amplitude"=w131, "damping"=w130) -> ("Upper Bound"=w134:dbl[], "Lower Bound"=w133:dbl[])  [unwired: 7 in, 3 out]
          }
          frame "Power" {
            n45 = call <vilib>:"Power Fit.vi"("Y"=w148, "X"=w147, "tolerance"=w149, "method"=w143) -> ("Best Power Fit"=w146:dbl[], "amplitude"=w141:dbl, "power"=w142:dbl, "residue"=w140:dbl)  [unwired: 6 in, 2 out]
            n46 = call-poly <vilib>:"Power Fit Intervals.vi"("Y"=w148, "X"=w147, "amplitude"=w141, "power"=w142) -> ("Upper Bound"=w145:dbl[], "Lower Bound"=w144:dbl[])  [unwired: 7 in, 3 out]
          }
          frame "Gaussian" {
            n47 = call <vilib>:"Gaussian Peak Fit.vi"("Y"=w153, "X"=w152, "tolerance"=w161, "method"=w157) -> ("Best Gaussian Fit"=w158:dbl[], "amplitude"=w154:dbl, "center"=w156:dbl, "standard deviation"=w155:dbl, "residue"=w151:dbl)  [unwired: 5 in, 2 out]
            n48 = call-poly <vilib>:"Gaussian Peak Fit Intervals.vi"("Y"=w153, "X"=w152, "amplitude"=w154, "center"=w156, "standard deviation"=w155) -> ("Upper Bound"=w160:dbl[], "Lower Bound"=w159:dbl[])  [unwired: 5 in, 4 out]
          }
          frame "Fit" {
          }
          frame "Logarithmic" {
            n49 = call <vilib>:"Logarithm Fit.vi"("Y"=w169, "X"=w167, "tolerance"=w168, "method"=w170) -> ("Best Logarithm Fit"=w171:dbl[], "amplitude"=w165:dbl, "scale"=w166:dbl, "residue"=w164:dbl)  [unwired: 7 in, 1 out]
            n50 = call-poly <vilib>:"Logarithm Fit Intervals.vi"("Y"=w169, "X"=w167, "amplitude"=w165, "scale"=w166) -> ("Upper Bound"=w172:dbl[], "Lower Bound"=w173:dbl[])  [unwired: 7 in, 3 out]
          }
        }
        "Slope Value" <- w96
        "Intercept Value" <- w95
        "Standard Deviation" <- w94
        "Residue" <- w90
        n51 = property on="Standard Deviation" class="DigNum (strict)"("Visible"=w87) -> ()  [unwired: 2 in, 2 out]
        n52 = case shown="0" "Fitting Method" {
          tunnel: w84 -> [w106 w113]
          tunnel: w85 -> [w101 w112]
          tunnel: w99 -> [w105 _]
          tunnel: w98 -> [w104 _]
          tunnel: w97 -> [w103 w114]
          tunnel: [w102 w111] -> w91
          frame 0 {
            # "Least squares"
            n53 = Build Cluster Array(w101, w106) -> (w108:cluster{"Numeric":dbl, "Numeric":dbl}[])
            n54 = Build Cluster Array(w101, w103) -> (w107:cluster{"Numeric":dbl, "Numeric":dbl}[])
            n55 = Build Cluster Array(w101, w104) -> (w110:cluster{"Numeric":dbl, "Numeric":dbl}[])
            n56 = Build Cluster Array(w101, w105) -> (w109:cluster{"Numeric":dbl, "Numeric":dbl}[])
            n57 = Build Cluster Array(w108, w107, w110, w109) -> (w102:T10)
          }
          frame 1, Default {
            # "Least absolute residual\nBi-square"
            n58 = Build Cluster Array(w112, w113) -> (w116:cluster{"Numeric":dbl, "Numeric":dbl}[])
            n59 = Build Cluster Array(w112, w114) -> (w115:cluster{"Numeric":dbl, "Numeric":dbl}[])
            n60 = Build Cluster Array(w116, w115) -> (w111:T10)
          }
        }
        "Observed Data and Fitted Curve" <- w91
        n61 = Wait (ms)(milliseconds to wait=u32 500) -> ()  [unwired: 1 out]
      }
    }
    frame Enabled {
      w176 = u16 0 items=["dB", "linear"] ("magnitude unit")
      n62 = call-poly <vilib>:"SI Estimate Transfer Function Model from FRF.vi"("FRF magnitude"=w182, "FRF phase"=w181, "orders of transfer function model"="orders of transfer function model", "sampling rate (Hz)"=12500.0) -> ("system model out"=w179:T5)  [unwired: 9 in, 2 out]
      n63 = call <vilib>:"SI Bode Plot.vi"("magnitude unit"=w176, "freq info"="freq info", "system model"=w179) -> ("Bode phase plot"=→"Bode phase plot":T1, "Bode magnitude plot"=→"Bode magnitude plot":T2)  [unwired: 6 in, 1 out]
    }
  }
